vi "总氮总磷质控流程.vi"(0 "队列输入TP":refnum<queue>, 5 "总氮量程切换":enum32{"H", "L", "AUTO"}(ring)=enum."AUTO", 7 "总磷量程切换":enum32{"H", "L", "AUTO"}(ring)=enum."AUTO", 9 "总磷":bool, 11 "总氮":bool) -> (4 "布尔":bool, 6 "总磷中断报警":bool, 8 "总氮中断报警":bool)   [LabVIEW 2016, in "质控单元.lvlib"]
panel:
  out "总磷":bool
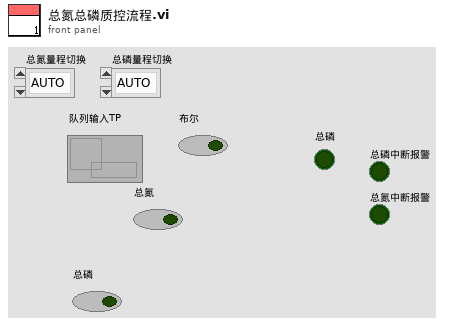
[diagram p1: front panel]
types:
  T1 = enum16{"待机", "启动氨氮水样", "氨氮测量中", "启动氨氮加标", "启动氨氮加标回收", "氨氮加标回收测量中", "启动总氮水样", "总氮测量中", "启动总氮加标", "启动总氮加标回收", "总氮加标回收测量中", "启动总磷水样", "总磷水样测量中", "启动总磷加标", "启动总磷加标回收", "总磷加标回收测量中", "结束"}
  T2 = cluster{"站号":u16, "量程切换":enum32{"H", "L", "AUTO"}, "控制命令":enum16{"启动测量", "标样核查", "零点核查", "跨度核查", "空白测试", "平行样测试", "加标回收", "空白校准", "标样校准", "初始化（清洗）", "停止测试", "仪器重启", "校时", "模式设置", "测量间隔设置"}, "模式设置":enum16{"待机", "连续模式", "周期模式", "定点模式", "受控模式", "手动模式"}, "测量间隔":u16}
  T3 = cluster{"时间标识":timestamp, "设备":string, "日志信息":string}
  T4 = cluster{"系统时间":timestamp, "工作状态":enum16{"空闲", "水样测试", "标样核查", "零点核查", "跨度核查", "空白测试", "平行样测试", "加标回收", "空白校准", "标样校准", "初始化（清洗）"}, "测量模式":enum16{"待机", "连续模式", "周期模式", "定点模式", "受控模式", "手动模式"}, "告警代码":enum16{"无告警", "缺试剂告警", "缺水样告警", "缺蒸馏水告警", "缺标液告警", "仪表漏液告警", "标定异常告警", "超量程告警", "加热异常", "低试剂预警", "超上限告警", "超下限告警", "仪表内部其他异常", "滴定异常告警", "电极异常告警", "量程切换告警", "参数设置告警", "PH电极电位异常", "电导率电极异常", "浊度光度异常", "溶解氧电极异常", "溶解氧光强异常", "温度异常告警", "PH异常告警", "溶解氧异常告警", "电导率异常告警", "浊度异常告警", "叶绿素异常告警", "藻密度异常告警", "蓝绿藻异常告警", "ORP异常告警", "氨氮异常告警", "清洁刷异常告警", "SD卡异常告警", "蓝牙异常告警", "Wifi异常告警", "流程异常告警"}, "故障代码":enum16{"无故障", "电机故障", "温度故障", "通讯故障", "滴定故障"}, "日志代码":u16, "软件版本":u16, "F0":sgl, "F1":sgl, "F2":sgl, "F3":sgl, "T":sgl, "H":sgl, "id":u16, "flowid":u16, "量程":u16, "总磷控温温度1":sgl, "营养盐控温温度2":sgl, "ADC":sgl}
  T5 = enum16{"空闲", "水样测试", "标样核查", "零点核查", "跨度核查", "空白测试", "平行样测试", "加标回收", "空白校准", "标样校准", "初始化（清洗）"}
  T6 = cluster{"因子编码":u32, "单位":u16, "标样参考值":sgl, "水样数据时间":timestamp, "水样实测值":sgl, "水样数据标识":string, "标样数据时间":timestamp, "标样实测值":sgl, "标样数据标识":string, "空白数据时间":timestamp, "空白实测值":sgl, "空白数据标识":string, "零点核查数据时间":timestamp, "零点核查实测值":sgl, "零点核查数据标识":string, "跨度核查数据时间":timestamp, "跨度核查实测值":sgl, "跨度核查数据标识":string, "加标回收数据时间":timestamp, "加标回收实测值":sgl, "加标回收数据标识":string, "平行样数据时间":timestamp, "平行样实测值":sgl, "平行样数据标识":string}
  T7 = cluster{"量程":dbl, "检出限":dbl, "加标前水样浓度":dbl, "加标后水样浓度":dbl, "加标水杯定容体积":dbl, "加标母液浓度":dbl, "加标体积":dbl, "加标回收率":dbl}
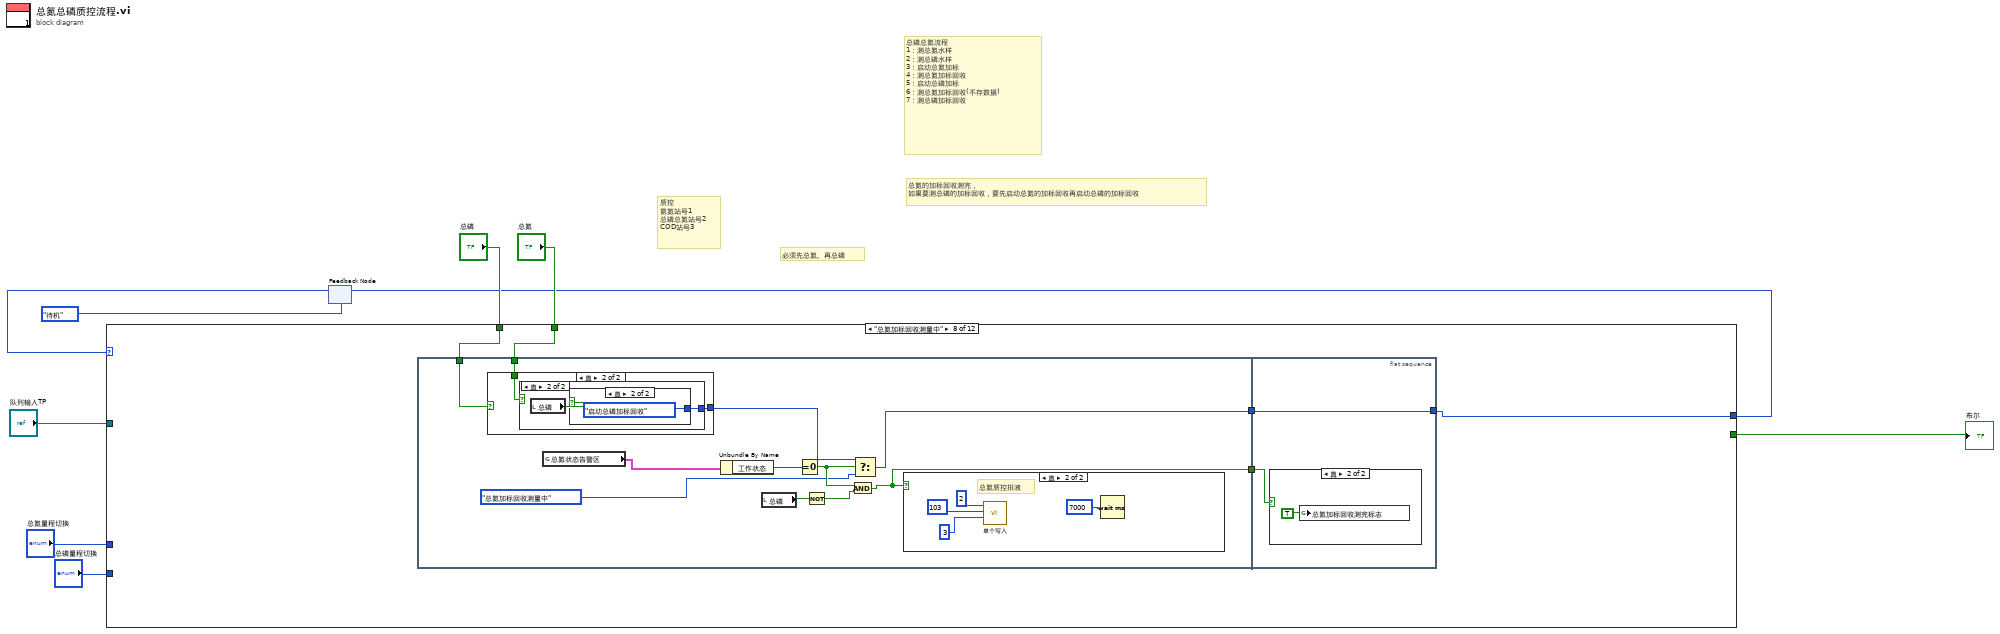
[diagram p0: block diagram]
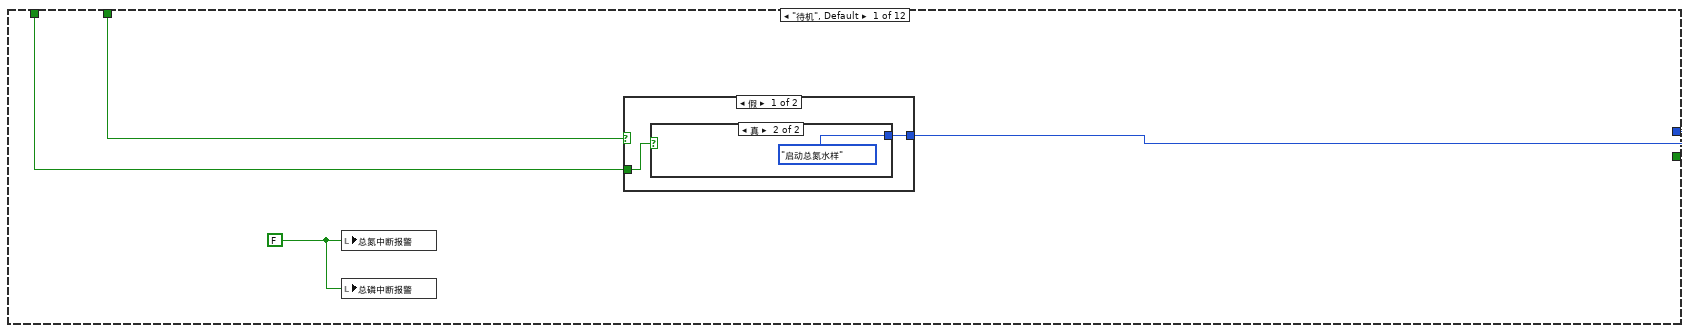
[diagram p2: hidden frame]
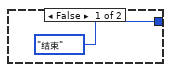
[diagram p3: hidden frame]
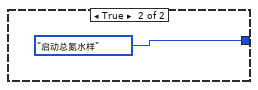
[diagram p4: hidden frame]
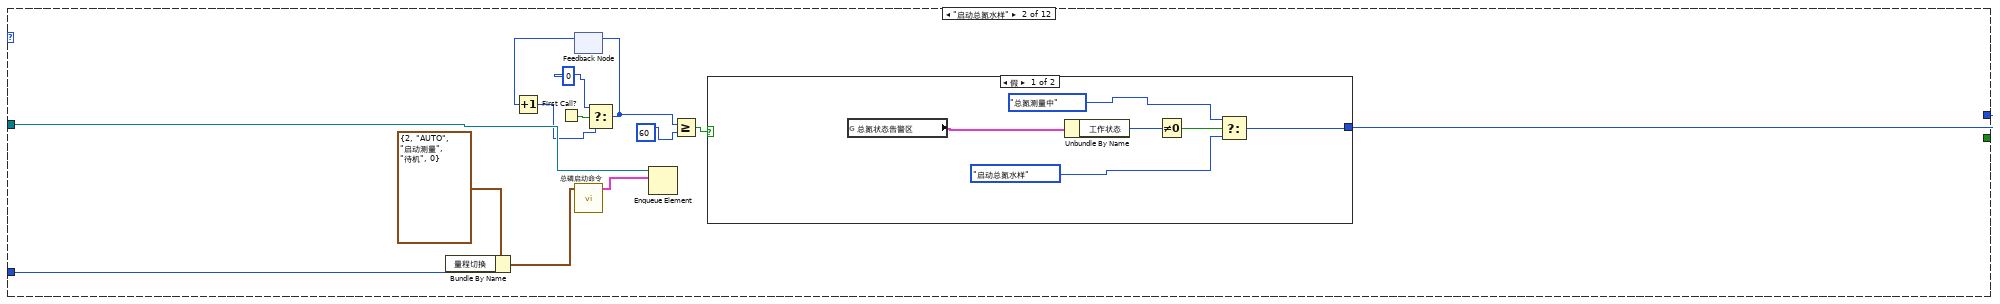
[diagram p5: hidden frame]
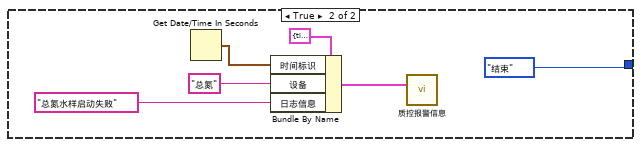
[diagram p6: hidden frame]
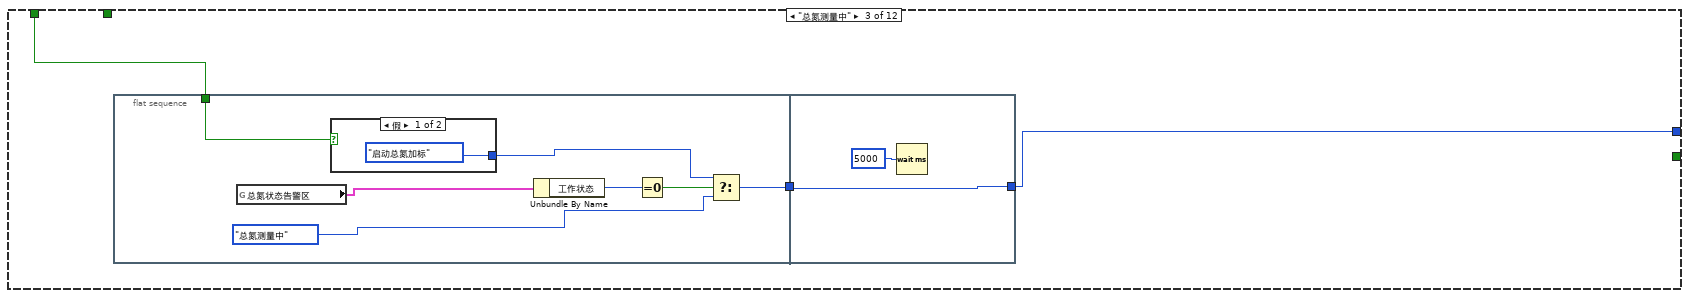
[diagram p7: hidden frame]
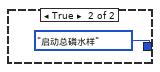
[diagram p8: hidden frame]
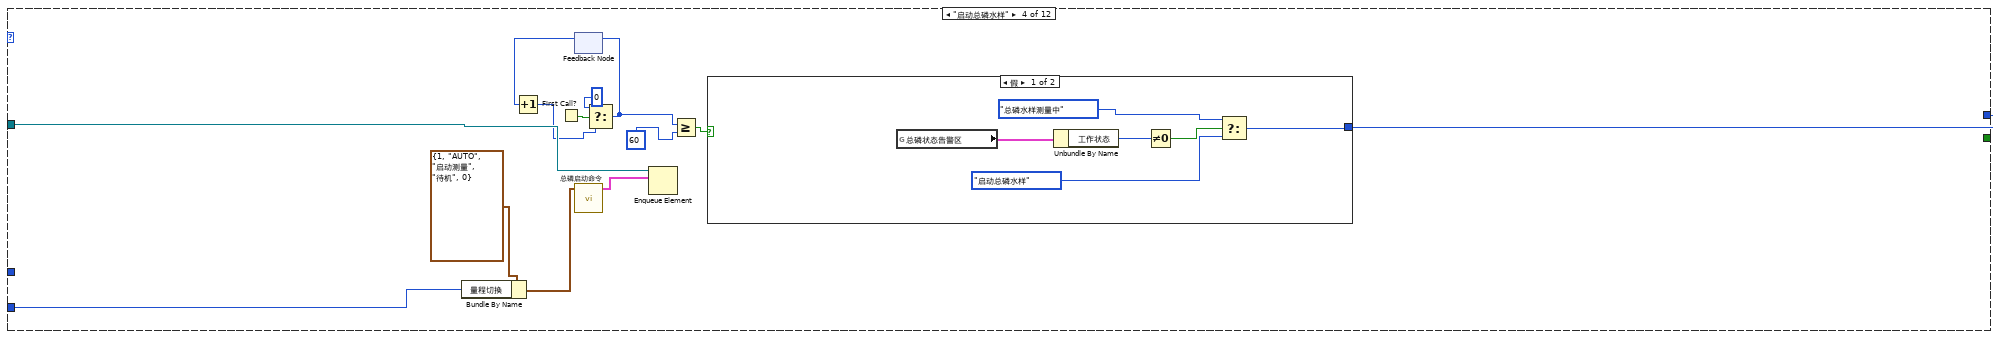
[diagram p9: hidden frame]
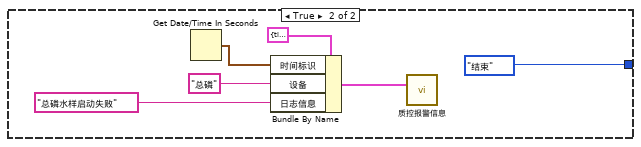
[diagram p10: hidden frame]
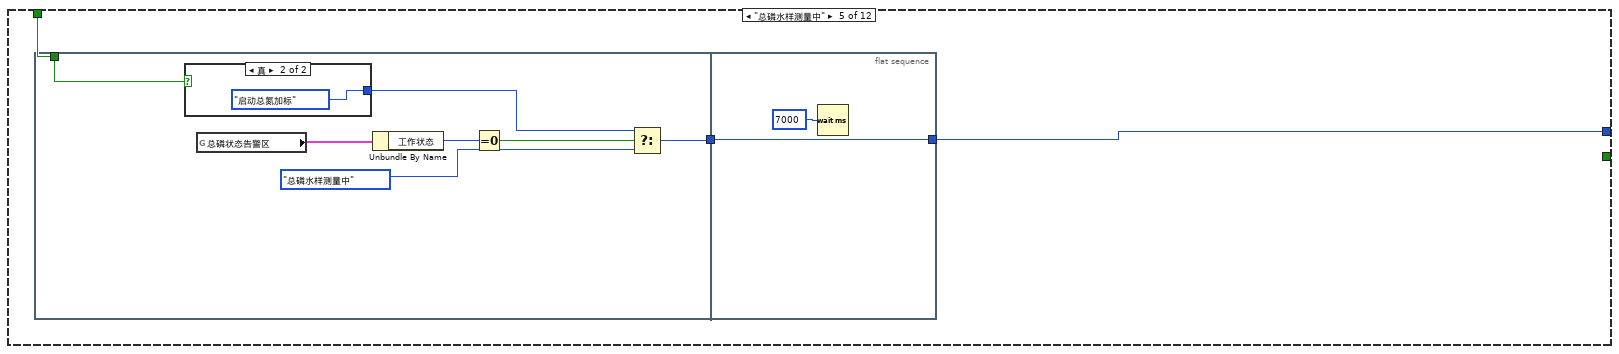
[diagram p11: hidden frame]
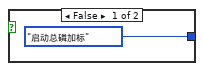
[diagram p12: hidden frame]
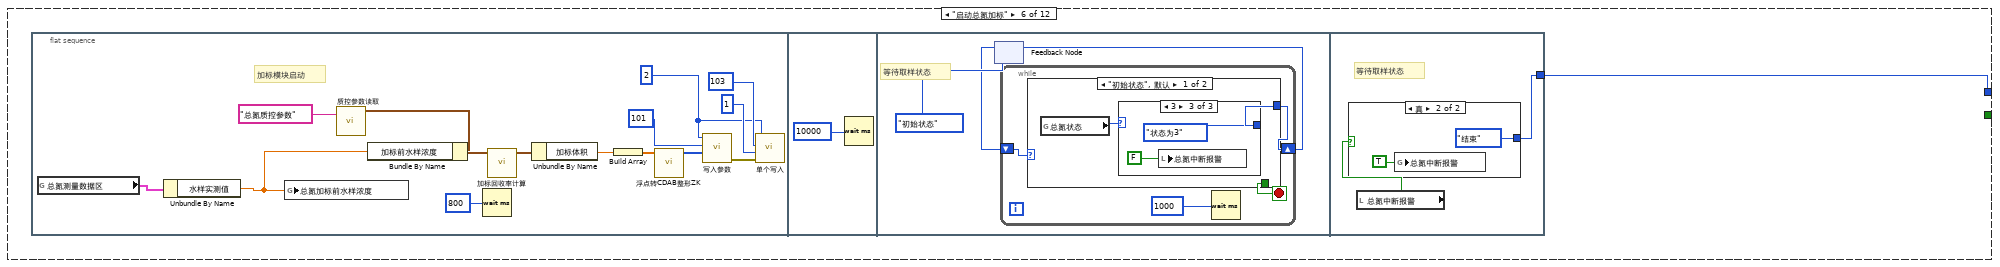
[diagram p13: hidden frame]
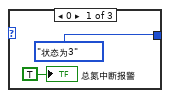
[diagram p14: hidden frame]
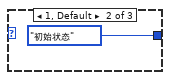
[diagram p15: hidden frame]
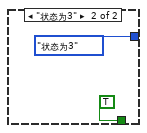
[diagram p16: hidden frame]
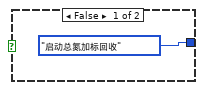
[diagram p17: hidden frame]
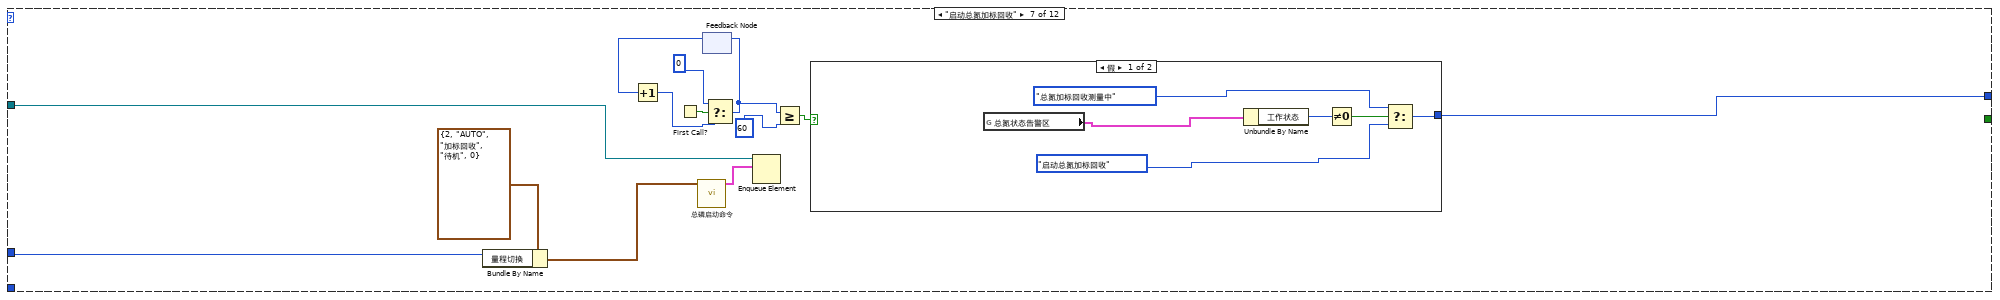
[diagram p18: hidden frame]
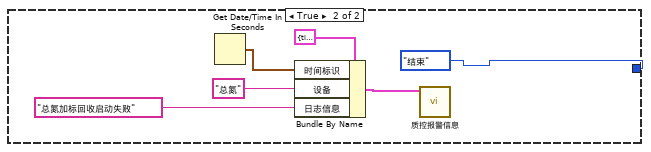
[diagram p19: hidden frame]
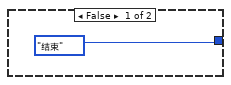
[diagram p20: hidden frame]
diagram:
  # "总磷总氮流程\n1：测总氮水样\n2：测总磷水样\n3：启动总氮加标\n4：测总氮加标回收\n5：启动总磷加标\n6：测总氮加标回收(不存数据)\n7：测总磷加标回收"
  # "总氮的加标回收测完，\n如果要测总磷的加标回收，要先启动总氮的加标回收再启动总磷的加标回收"
  # "质控\n氨氮站号1   \n总磷总氮站号2\nCOD站号3"
  # "必须先总氮、再总磷"
  n1 = feedback #1(T1."待机") -> (w5:T1)
  n2 = case shown="\"总氮加标回收测量中\"" w5 {
    tunnel: [w13 w30 w45 w69 w85 w97 w138 w162 w191 w235 w258 T1."结束"] -> w3
    tunnel: "队列输入TP" -> [_ w31 _ w70 _ _ w140 _ _ w236 _ _]
    tunnel: [_ _ _ _ _ _ _ _ _ _ _ TRUE] -> w8
    tunnel: "总磷" -> [w12 _ w44 _ _ _ _ w163 _ _ _ _]
    tunnel: "总氮" -> [w11 _ _ _ w83 _ _ w161 _ _ _ _]
    tunnel: "总氮量程切换" -> [_ w19 _ _ _ _ w135 _ _ _ _ _]
    tunnel: "总磷量程切换" -> [_ _ _ w58 _ _ _ _ _ w231 _ _]
    frame "待机", Default {
      w10 = FALSE ("总氮中断报警")
      n3 = local write "总氮中断报警"(w10) -> ()
      n4 = local write "总磷中断报警"(w10) -> ()
      n5 = case shown="假" w11 {
        tunnel: w12 -> [w14 _]
        tunnel: [w15 T1."启动总氮水样"] -> w13
        frame False {
          n6 = case shown="真" w14 {
            tunnel: [T1."结束" T1."启动总氮水样"] -> w15
            frame False {
            }
            frame True {
            }
          }
        }
        frame True {
        }
      }
    }
    frame "启动总氮水样" {
      n7 = Bundle By Name(cluster=T2 {"站号"=2, "量程切换"=enum."AUTO", "控制命令"=enum."启动测量", "模式设置"=enum."待机", "测量间隔"=0} ("参数"), "量程切换"=w19) -> (w20:T2)
      n8 = First Call?() -> (First Call?: T/F=w28:bool)
      n9 = feedback #2() -> (w27:i32)  [unwired: 1 in]
      n10 = Increment(x=w27) -> (x+1=w26:i32)
      n11 = call "总磷启动命令.vi"("参数"=w20) -> ("启动命令"=w22:cluster{"命令":string, "data":variant})  [unwired: 10 in]
      n12 = Select(t=0, s=w28, f=w26) -> (s? t:f=w25:i32)
      n13 = feedback-in #2(w25) -> ()
      n14 = Enqueue Element(queue=w31, element=w22) -> ()  [unwired: 2 in, 3 out]
      n15 = Greater Or Equal?(x=w25, y=60) -> (x >= y?=w23:bool)
      n16 = case shown="假" w23 {
        tunnel: [w35 T1."结束"] -> w30
        frame False {
          n17 = global read "与总氮交互全局.vi" "总氮状态告警区"() -> (w32:T4)
          n18 = Unbundle By Name(w32) -> ("工作状态"=w36:T5)
          n19 = Not Equal To 0?(x=w36) -> (x != 0?=w37:bool)
          n20 = Select(t=T1."总氮测量中", s=w37, f=T1."启动总氮水样") -> (s? t:f=w35:T1)
        }
        frame True {
          n21 = Get Date/Time In Seconds() -> (seconds since 1Jan1904=w43:timestamp)
          n22 = Bundle By Name(cluster=T3 {"时间标识"=timestamp(0 s since 1904-01-01), "设备"="", "日志信息"=""} ("data in"), "时间标识"=w43, "设备"="总氮", "日志信息"="总氮水样启动失败") -> (w39:T3)
          n23 = call "质控报警信息.vi"("data in"=w39) -> ()  [unwired: 11 in]
        }
      }
    }
    frame "总氮测量中" {
      n24 = flat-sequence {
        tunnel: [w52] -> w46
        tunnel: w44 -> [w48]
        tunnel: [w57] -> w45
        tunnel: w46 -> [w57]
        frame #0 {
          n25 = global read "与总氮交互全局.vi" "总氮状态告警区"() -> (w47:T4)
          n26 = case shown="假" w48 {
            tunnel: [T1."启动总氮加标" T1."启动总磷水样"] -> w50
            frame False {
            }
            frame True {
            }
          }
          n27 = Unbundle By Name(w47) -> ("工作状态"=w53:T5)
          n28 = Equal To 0?(x=w53) -> (x = 0?=w51:bool)
          n29 = Select(t=w50, s=w51, f=T1."总氮测量中") -> (s? t:f=w52:T1)
        }
        frame #1 {
          n30 = Wait (ms)(milliseconds to wait=u32 5000 ("等待时间（毫秒）")) -> ()  [unwired: 1 out]
        }
      }
    }
    frame "启动总磷水样" {
      n31 = Bundle By Name(cluster=T2 {"站号"=1, "量程切换"=enum."AUTO", "控制命令"=enum."启动测量", "模式设置"=enum."待机", "测量间隔"=0} ("参数"), "量程切换"=w58) -> (w59:T2)
      n32 = First Call?() -> (First Call?: T/F=w67:bool)
      n33 = feedback #3() -> (w66:i32)  [unwired: 1 in]
      n34 = Increment(x=w66) -> (x+1=w65:i32)
      n35 = call "总磷启动命令.vi"("参数"=w59) -> ("启动命令"=w61:cluster{"命令":string, "data":variant})  [unwired: 10 in]
      n36 = Select(t=0, s=w67, f=w65) -> (s? t:f=w64:i32)
      n37 = feedback-in #3(w64) -> ()
      n38 = Enqueue Element(queue=w70, element=w61) -> ()  [unwired: 2 in, 3 out]
      n39 = Greater Or Equal?(x=w64, y=60) -> (x >= y?=w62:bool)
      n40 = case shown="假" w62 {
        tunnel: [w73 T1."结束"] -> w69
        frame False {
          n41 = global read "与总磷交互全局.vi" "总磷状态告警区"() -> (w74:T4)
          n42 = Unbundle By Name(w74) -> ("工作状态"=w75:T5)
          n43 = Not Equal To 0?(x=w75) -> (x != 0?=w76:bool)
          n44 = Select(t=T1."总磷水样测量中", s=w76, f=T1."启动总磷水样") -> (s? t:f=w73:T1)
        }
        frame True {
          n45 = Get Date/Time In Seconds() -> (seconds since 1Jan1904=w82:timestamp)
          n46 = Bundle By Name(cluster=T3 {"时间标识"=timestamp(0 s since 1904-01-01), "设备"="", "日志信息"=""} ("data in"), "时间标识"=w82, "设备"="总磷", "日志信息"="总磷水样启动失败") -> (w78:T3)
          n47 = call "质控报警信息.vi"("data in"=w78) -> ()  [unwired: 11 in]
        }
      }
    }
    frame "总磷水样测量中" {
      n48 = flat-sequence {
        tunnel: [w90] -> w84
        tunnel: w83 -> [w87]
        tunnel: [w96] -> w85
        tunnel: w84 -> [w96]
        frame #0 {
          n49 = case shown="真" w87 {
            tunnel: [T1."启动总磷加标" T1."启动总氮加标"] -> w88
            frame False {
            }
            frame True {
            }
          }
          n50 = global read "与总磷交互全局.vi" "总磷状态告警区"() -> (w91:T4)
          n51 = Unbundle By Name(w91) -> ("工作状态"=w92:T5)
          n52 = Equal To 0?(x=w92) -> (x = 0?=w89:bool)
          n53 = Select(t=w88, s=w89, f=T1."总磷水样测量中") -> (s? t:f=w90:T1)
        }
        frame #1 {
          n54 = Wait (ms)(milliseconds to wait=u32 7000 ("等待时间（毫秒）")) -> ()  [unwired: 1 out]
        }
      }
    }
    frame "启动总氮加标" {
      n55 = flat-sequence {
        tunnel: [w131] -> w97
        frame #0 {
          w99 = u16 2 ("value")
          # "加标模块启动"
          n56 = global read "与总氮交互全局.vi" "总氮测量数据区"() -> (w98:T6)
          n57 = Unbundle By Name(w98) -> ("水样实测值"=w100:sgl)
          n58 = global write "水样浓度全局.vi" "总氮加标前水样浓度"(w100) -> ()
          n59 = call "质控参数读取.vi"("section"="总氮质控参数") -> ("参数"=w102:T7)  [unwired: 9 in, 1 out]
          n60 = Bundle By Name(cluster=w102, "加标前水样浓度"=w100) -> (w111:T7)
          n61 = Wait (ms)(milliseconds to wait=u32 800 ("等待时间（毫秒）")) -> ()  [unwired: 1 out]
          n62 = call "加标回收率计算.vi"("参数"=w111) -> ("参数 out"=w110:T7)  [unwired: 10 in]
          n63 = Unbundle By Name(w110) -> ("加标体积"=w103:dbl)
          n64 = Build Array(w103) -> (w109:dbl[])
          n65 = call "浮点转CDAB整形ZK.vi"("浮点数"=w109) -> ("CDAB整形输出"=w104:u16[])  [unwired: 10 in]
          n66 = call "写入参数.vi"("values"=w104, "starting address"=u16 101, "Slave ID"=w99) -> ("error out"=w108:errorcluster)  [unwired: 8 in]
          n67 = call "单个写入.vi"("Error in"=w108, "value"=u16 1, "address"=u16 103, "Slave ID"=w99) -> ()  [unwired: 7 in, 1 out]
        }
        frame #1 {
          n68 = Wait (ms)(milliseconds to wait=u32 10000 ("等待时间（毫秒）")) -> ()  [unwired: 1 out]
        }
        frame #2 {
          # "等待取样状态"
          n69 = feedback #4(enum16{"初始状态", "状态为3"}."初始状态") -> (w115:enum16{"初始状态", "状态为3"})
          n70 = while {
            shift-right: [w119] -> w114
            shift-left: w115 -> [w120]
            stop <- w118 stop-if-true
            n71 = case shown="\"初始状态\", 默认" w120 {
              tunnel: [w122 enum16{"初始状态", "状态为3"}."状态为3"] -> w119
              tunnel: [_ TRUE] -> w118
              frame "初始状态", Default {
                n72 = global read "加标回收状态全局变量.vi" "总氮状态"() -> (w121:u16)
                n73 = case shown="3" w121 {
                  tunnel: [enum16{"初始状态", "状态为3"}."状态为3" enum16{"初始状态", "状态为3"}."初始状态" enum16{"初始状态", "状态为3"}."状态为3"] -> w122
                  frame 0 {
                    "总氮中断报警" <- TRUE ("总氮中断报警")
                  }
                  frame 1, Default {
                  }
                  frame 3 {
                    n74 = local write "总氮中断报警"(FALSE ("总氮中断报警")) -> ()
                  }
                }
              }
              frame "状态为3" {
              }
            }
            n75 = Wait (ms)(milliseconds to wait=u32 1000 ("等待时间（毫秒）")) -> ()  [unwired: 1 out]
          }
          n76 = feedback-in #4(w114) -> ()
        }
        frame #3 {
          # "等待取样状态"
          n77 = local read "总氮中断报警"() -> (w130:bool)
          n78 = case shown="真" w130 {
            tunnel: [T1."启动总氮加标回收" T1."结束"] -> w131
            frame False {
            }
            frame True {
              n79 = global write "质控中断报警全局.vi" "总氮中断报警"(TRUE ("总氮中断报警")) -> ()
            }
          }
        }
      }
    }
    frame "启动总氮加标回收" {
      n80 = Bundle By Name(cluster=T2 {"站号"=2, "量程切换"=enum."AUTO", "控制命令"=enum."加标回收", "模式设置"=enum."待机", "测量间隔"=0} ("参数"), "量程切换"=w135) -> (w136:T2)
      n81 = First Call?() -> (First Call?: T/F=w146:bool)
      n82 = call "总磷启动命令.vi"("参数"=w136) -> ("启动命令"=w139:cluster{"命令":string, "data":variant})  [unwired: 10 in]
      n83 = feedback #5() -> (w145:i32)  [unwired: 1 in]
      n84 = Increment(x=w145) -> (x+1=w144:i32)
      n85 = Select(t=0, s=w146, f=w144) -> (s? t:f=w143:i32)
      n86 = feedback-in #5(w143) -> ()
      n87 = Enqueue Element(queue=w140, element=w139) -> ()  [unwired: 2 in, 3 out]
      n88 = Greater Or Equal?(x=w143, y=60) -> (x >= y?=w141:bool)
      n89 = case shown="假" w141 {
        tunnel: [w151 T1."结束"] -> w138
        frame False {
          n90 = global read "与总氮交互全局.vi" "总氮状态告警区"() -> (w148:T4)
          n91 = Unbundle By Name(w148) -> ("工作状态"=w153:T5)
          n92 = Not Equal To 0?(x=w153) -> (x != 0?=w152:bool)
          n93 = Select(t=T1."总氮加标回收测量中", s=w152, f=T1."启动总氮加标回收") -> (s? t:f=w151:T1)
        }
        frame True {
          n94 = Get Date/Time In Seconds() -> (seconds since 1Jan1904=w159:timestamp)
          n95 = Bundle By Name(cluster=T3 {"时间标识"=timestamp(0 s since 1904-01-01), "设备"="", "日志信息"=""} ("data in"), "时间标识"=w159, "设备"="总氮", "日志信息"="总氮加标回收启动失败") -> (w155:T3)
          n96 = call "质控报警信息.vi"("data in"=w155) -> ()  [unwired: 11 in]
        }
      }
    }
    frame "总氮加标回收测量中" {
      n97 = flat-sequence {
        tunnel: [w174] -> w164
        tunnel: w163 -> [w171]
        tunnel: w161 -> [w167]
        tunnel: [w165] -> w160
        tunnel: [w189] -> w162
        tunnel: w164 -> [w189]
        tunnel: w160 -> [w188]
        frame #0 {
          n98 = case shown="真" w171 {
            tunnel: [T1."结束" w178] -> w173
            tunnel: w167 -> [_ w177]
            frame False {
            }
            frame True {
              n99 = case shown="真" w177 {
                tunnel: [T1."启动总磷加标回收" w181] -> w178
                frame False {
                }
                frame True {
                  n100 = local read "总磷"() -> (w180:bool)
                  n101 = case shown="真" w180 {
                    tunnel: [T1."启动总磷加标" T1."启动总磷加标回收"] -> w181
                    frame False {
                    }
                    frame True {
                    }
                  }
                }
              }
            }
          }
          n102 = global read "与总氮交互全局.vi" "总氮状态告警区"() -> (w166:T4)
          n103 = Unbundle By Name(w166) -> ("工作状态"=w175:T5)
          n104 = local read "总磷"() -> (w169:bool)
          n105 = Equal To 0?(x=w175) -> (x = 0?=w172:bool)
          n106 = Not(x=w169) -> (.not. x?=w168:bool)
          n107 = And(x=w172, y=w168) -> (x .and. y?=w165:bool)
          n108 = Select(t=w173, s=w172, f=T1."总氮加标回收测量中") -> (s? t:f=w174:T1)
          n109 = case shown="真" w165 {
            frame False {
            }
            frame True {
              # "总氮质控排液"
              n110 = call "单个写入.vi"("value"=u16 3, "address"=u16 103, "Slave ID"=u8 2) -> ()  [unwired: 8 in, 1 out]
              n111 = Wait (ms)(milliseconds to wait=u32 7000 ("等待时间（毫秒）")) -> ()  [unwired: 1 out]
            }
          }
        }
        frame #1 {
          n112 = case shown="真" w188 {
            frame False {
            }
            frame True {
              n113 = global write "质控测完标志全局 1.vi" "总氮加标回收测完标志"(TRUE) -> ()
            }
          }
        }
      }
    }
    frame "启动总磷加标" {
      n114 = flat-sequence {
        tunnel: [w227] -> w191
        frame #0 {
          n115 = Wait (ms)(milliseconds to wait=u32 180000 ("等待时间（毫秒）")) -> ()  [unwired: 1 out]
        }
        frame #1 {
          w198 = u16 2 ("value")
          # "加标模块启动"
          n116 = global read "与总磷交互全局.vi" "总磷测量数据区"() -> (w194:T6)
          n117 = Unbundle By Name(w194) -> ("水样实测值"=w193:sgl)
          n118 = call "质控参数读取.vi"("section"="总磷质控参数") -> ("参数"=w196:T7)  [unwired: 9 in, 1 out]
          n119 = Bundle By Name(cluster=w196, "加标前水样浓度"=w193) -> (w206:T7)
          n120 = global write "水样浓度全局.vi" "总磷加标前水样浓度"(w193) -> ()
          n121 = Wait (ms)(milliseconds to wait=u32 800 ("等待时间（毫秒）")) -> ()  [unwired: 1 out]
          n122 = call "加标回收率计算.vi"("参数"=w206) -> ("参数 out"=w205:T7)  [unwired: 10 in]
          n123 = Unbundle By Name(w205) -> ("加标体积"=w197:dbl)
          n124 = Build Array(w197) -> (w204:dbl[])
          n125 = call "浮点转CDAB整形ZK.vi"("浮点数"=w204) -> ("CDAB整形输出"=w199:u16[])  [unwired: 10 in]
          n126 = call "写入参数.vi"("values"=w199, "starting address"=u16 101, "Slave ID"=w198) -> ("error out"=w203:errorcluster)  [unwired: 8 in]
          n127 = call "单个写入.vi"("Error in"=w203, "value"=u16 1, "address"=u16 103, "Slave ID"=w198) -> ()  [unwired: 7 in, 1 out]
        }
        frame #2 {
          n128 = Wait (ms)(milliseconds to wait=u32 10000 ("等待时间（毫秒）")) -> ()  [unwired: 1 out]
        }
        frame #3 {
          # "等待取样状态"
          n129 = feedback #6(enum16{"初始状态", "状态为3"}."初始状态") -> (w210:enum16{"初始状态", "状态为3"})
          n130 = while {
            shift-right: [w214] -> w209
            shift-left: w210 -> [w215]
            stop <- w213 stop-if-true
            n131 = case shown="\"状态为3\"" w215 {
              tunnel: [w217 enum16{"初始状态", "状态为3"}."状态为3"] -> w214
              tunnel: [_ TRUE] -> w213
              frame "初始状态", Default {
                n132 = global read "加标回收状态全局变量.vi" "总磷状态"() -> (w216:u16)
                n133 = case shown="0" w216 {
                  tunnel: [enum16{"初始状态", "状态为3"}."状态为3" enum16{"初始状态", "状态为3"}."初始状态" enum16{"初始状态", "状态为3"}."状态为3"] -> w217
                  frame 0 {
                    "总磷中断报警" <- TRUE ("总磷中断报警")
                  }
                  frame 1, Default {
                  }
                  frame 3 {
                    n134 = local write "总磷中断报警"(FALSE ("总磷中断报警")) -> ()
                  }
                }
              }
              frame "状态为3" {
                "总磷" <- TRUE
              }
            }
            n135 = Wait (ms)(milliseconds to wait=u32 1000 ("等待时间（毫秒）")) -> ()  [unwired: 1 out]
          }
          n136 = feedback-in #6(w209) -> ()
        }
        frame #4 {
          n137 = local read "总磷中断报警"() -> (w226:bool)
          n138 = case shown="真" w226 {
            tunnel: [T1."启动总氮加标回收" T1."结束"] -> w227
            frame False {
              # "等待取样状态"
            }
            frame True {
              n139 = global write "质控中断报警全局.vi" "总磷中断报警"(TRUE ("总磷中断报警")) -> ()
            }
          }
        }
      }
    }
    frame "启动总磷加标回收" {
      n140 = Bundle By Name(cluster=T2 {"站号"=1, "量程切换"=enum."AUTO", "控制命令"=enum."加标回收", "模式设置"=enum."待机", "测量间隔"=0} ("参数"), "量程切换"=w231) -> (w232:T2)
      n141 = First Call?() -> (First Call?: T/F=w243:bool)
      n142 = feedback #7() -> (w242:i32)  [unwired: 1 in]
      n143 = Increment(x=w242) -> (x+1=w241:i32)
      n144 = call "总磷启动命令.vi"("参数"=w232) -> ("启动命令"=w237:cluster{"命令":string, "data":variant})  [unwired: 10 in]
      n145 = Select(t=0, s=w243, f=w241) -> (s? t:f=w240:i32)
      n146 = feedback-in #7(w240) -> ()
      n147 = Enqueue Element(queue=w236, element=w237) -> ()  [unwired: 2 in, 3 out]
      n148 = Greater Or Equal?(x=w240, y=60) -> (x >= y?=w238:bool)
      n149 = case shown="真" w238 {
        tunnel: [w247 T1."结束"] -> w235
        frame False {
          n150 = global read "与总磷交互全局.vi" "总磷状态告警区"() -> (w248:T4)
          n151 = Unbundle By Name(w248) -> ("工作状态"=w249:T5)
          n152 = Not Equal To 0?(x=w249) -> (x != 0?=w250:bool)
          n153 = Select(t=T1."总磷加标回收测量中", s=w250, f=T1."启动总磷加标回收") -> (s? t:f=w247:T1)
        }
        frame True {
          n154 = Get Date/Time In Seconds() -> (seconds since 1Jan1904=w256:timestamp)
          n155 = Bundle By Name(cluster=T3 {"时间标识"=timestamp(0 s since 1904-01-01), "设备"="", "日志信息"=""} ("data in"), "时间标识"=w256, "设备"="总磷", "日志信息"="总磷加标回收启动失败") -> (w252:T3)
          n156 = call "质控报警信息.vi"("data in"=w252) -> ()  [unwired: 11 in]
        }
      }
      n157 = local write "总磷"(FALSE ("总磷")) -> ()
    }
    frame "总磷加标回收测量中" {
      n158 = flat-sequence {
        tunnel: [w263] -> w259
        tunnel: [w260] -> w257
        tunnel: [w271] -> w258
        tunnel: w259 -> [w271]
        tunnel: w257 -> [w270]
        frame #0 {
          n159 = global read "与总磷交互全局.vi" "总磷状态告警区"() -> (w264:T4)
          n160 = Unbundle By Name(w264) -> ("工作状态"=w265:T5)
          n161 = Equal To 0?(x=w265) -> (x = 0?=w260:bool)
          n162 = Select(t=T1."结束", s=w260, f=T1."总磷加标回收测量中") -> (s? t:f=w263:T1)
          n163 = case shown="真" w260 {
            frame False {
            }
            frame True {
              # "总磷质控排液"
              n164 = Wait (ms)(milliseconds to wait=u32 5000 ("等待时间（毫秒）")) -> ()  [unwired: 1 out]
              n165 = call "单个写入.vi"("value"=u16 3, "address"=u16 103, "Slave ID"=u8 2) -> ()  [unwired: 8 in, 1 out]
            }
          }
        }
        frame #1 {
          n166 = case shown="真" w270 {
            frame False {
            }
            frame True {
              n167 = global write "质控测完标志全局 1.vi" "总磷加标回收测完标志"(TRUE) -> ()
            }
          }
        }
      }
    }
    frame "结束" {
      n168 = Wait (ms)(milliseconds to wait=u32 5000 ("等待时间（毫秒）")) -> ()  [unwired: 1 out]
    }
  }
  "布尔" <- w8
  n169 = feedback-in #1(w3) -> ()
